vi "Create.vi"(7 "Shared Resource (F)":bool, 8 "error in (no error)":errorcluster, 10 "Subsystem Name (optional)":string, 11 "SMO":refnum<class "SMO.lvclass">) -> (0 "error out":errorcluster, 2 "SMO name":string, 3 "SMO out":refnum<class "SMO.lvclass">)   [LabVIEW 2021, in "smo.lvlib" / "SMO.lvclass"]
doc: "This method is called to create a new SMO instance.\n\n\"Subsystem name\" is a plain text name that this SMO instance will be registered with.\nIt is used in the inheritance hierarchy and stored in the Lineage attribute. The subsystem name must be unique in the dependence tree (i.e uniquely named if more than one susbystsms have the same owner). Empty spaces will be replaced by underscores. Avoid using dot notation in the subsystem's name if you intend to use the lineage to make this subsystem addressable through dot notation.\n\n\"Shared Resource (F)\" default to FALSE and determines whether the subsystem can be found by other SMOs for aggregation as a resource that is shared between multiple subsystems. An example would be a camera that can be used as a barcode reader by a module, or as an analytic sensor by another.\n\n\"SMO name\" is the unique name given to a subsystem. If the name is already taken, _%04d is appended to the input name."
uses:
  SMO.lvclass
  Typedefs/SMOState --Enum.ctl
  SMO.lvclass/SMO.ctl
panel:
  # "For instructions on how to use the JKI State Machine Objects, examples and video tutorials, visit:\nhttp://jki.net/state-machine-objects/\n\nJKI State Machine Objects™\nhttp://jki.net/state-machine-objects/\nCopyright (C) 2005-2015, JKI <info@jki.net>\nALL RIGHTS RESERVED"
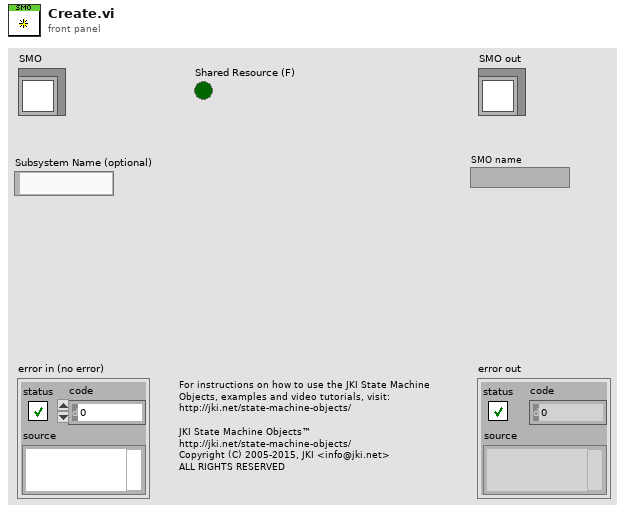
[diagram p1: front panel]
types:
  T1 = typedef "smo.lvlib/SMO.lvclass/SMOState --Enum.ctl" = enum16{"unknown", "Created", "Started", "Stopped"}
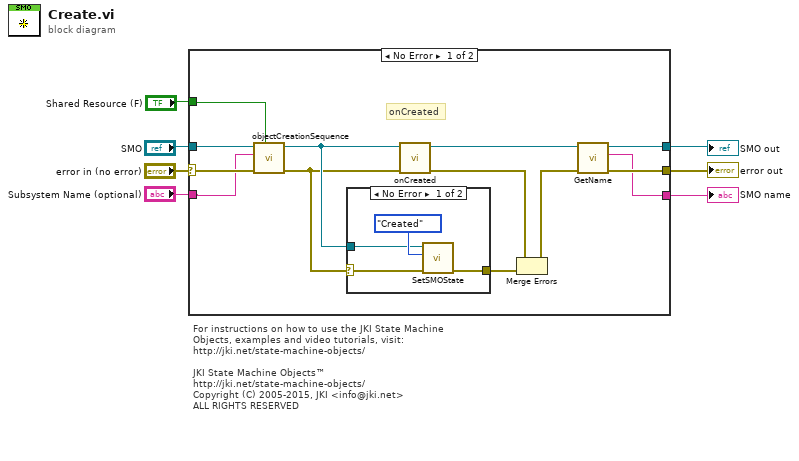
[diagram p0: block diagram]
diagram:
  # "For instructions on how to use the JKI State Machine Objects, examples and video tutorials, visit:\nhttp://jki.net/state-machine-objects/\n\nJKI State Machine Objects™\nhttp://jki.net/state-machine-objects/\nCopyright (C) 2005-2015, JKI <info@jki.net>\nALL RIGHTS RESERVED"
  n1 = case shown="No Error" "error in (no error)" {
    selector: "error in (no error)" -> [w19 w27]
    tunnel: [w10 w27] -> w2
    tunnel: [w9 w26] -> w3
    tunnel: "SMO" -> [w20 w26]
    tunnel: "Subsystem Name (optional)" -> [w18 _]
    tunnel: [w8 _] -> w1
    tunnel: "Shared Resource (F)" -> [w17 _]
    frame No Error {
      # "onCreated"
      n2 = call "objectCreationSequence.vi"("Shared Resource (F)"=w17, "error in (no error)"=w19, "Subsystem Name (optional)"=w18, "SMO in"=w20) -> ("error out"=w15:errorcluster, "SMO out"=w16:refnum<class "SMO.lvclass">)  [unwired: 6 in]
      n3 = case shown="No Error" w15 {
        selector: w15 -> [w21 w25]
        tunnel: [w23 w25] -> w14
        tunnel: w16 -> [w22 _]
        frame No Error {
          n4 = call "SetSMOState.vi"("error in (no error)"=w21, "SMO State"=SMOState_--Enum."Created" ("event data"), "SMO in"=w22) -> ("error out"=w23:errorcluster)  [unwired: 7 in, 1 out]
        }
        frame Error {
        }
      }
      n5 = call-dynamic "onCreated.vi"("error in (no error)"=w15, "SMO"=w16) -> ("error out"=w13:errorcluster, "SMO out"=w12:refnum<class "SMO.lvclass">)  [unwired: 8 in]
      n6 = Merge Errors(w13, w14) -> (w11:errorcluster)
      n7 = call "GetName.vi"("error in (no error)"=w11, "SMO"=w12) -> ("error out"=w10:errorcluster, "Name"=w8:string, "SMO out"=w9:refnum<class "SMO.lvclass">)  [unwired: 6 in, 1 out]
    }
    frame Error {
    }
  }
  "error out" <- w2
  "SMO out" <- w3
  "SMO name" <- w1
